vi "ReadMaxAmp.vi"(8 "error in (no error)":errorcluster, 9 "Channel":dbl, 11 "Simulated Scope in":refnum<class "Simulated Scope.lvclass">) -> (0 "error out":errorcluster, 1 "Amplitude":dbl, 3 "Simulated Scope out":refnum<class "Simulated Scope.lvclass">)   [LabVIEW 2010, in "Simulated Scope.lvclass"]
uses:
  Simulated Scope.lvclass
  Simulated Scope Operation.ctl
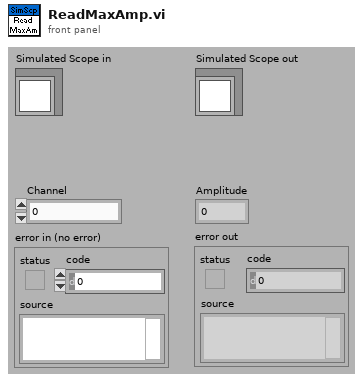
[diagram p1: front panel]
types:
  T1 = typedef "Simulated Scope.lvclass/Simulated Scope Operation.ctl" = enum16{"Read", "Clear"}
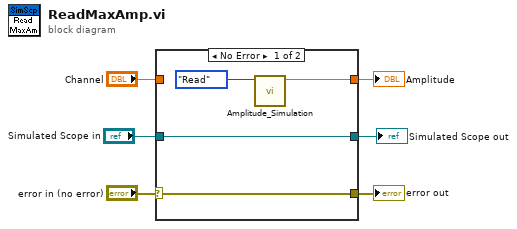
[diagram p0: block diagram]
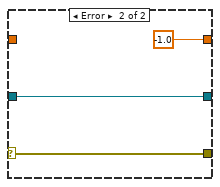
[diagram p2: hidden frame]
diagram:
  n1 = case shown="No Error" "error in (no error)" {
    selector: "error in (no error)" -> [w9 w12]
    tunnel: "Simulated Scope in" -> [w10 w13]
    tunnel: [w10 w13] -> w6
    tunnel: [w9 w12] -> w1
    tunnel: [w8 -1.0] -> w4
    tunnel: "Channel" -> [_ _]
    frame No Error {
      n2 = call "Amplitude_Simulation.vi"("Sim Scope Operation"=Simulated_Scope_Operation."Read") -> ("Amplitude"=w8:dbl)  [unwired: 10 out]
    }
    frame Error {
    }
  }
  "Simulated Scope out" <- w6
  "error out" <- w1
  "Amplitude" <- w4
